vi "Image_processor.vi"(6 "DUT":u16, 9 "Ref Folder":path, 10 "DUT_Conf":string="RX-DUT", 11 "Image Path":path) -> (2 "Fail_Strings":string, 3 "PASS/FAIL":bool)   [LabVIEW 2024, in "Keyence_VS150.lvlib"]
uses:
  Keyence_VS150.lvlib
  Image_match_details.ctl
  <vilib>/Utility/file.llb/Read Delimited Spreadsheet (string).vi
  Launcher/Launcher_DTU.lvlib
panel:
  out "Array 3":T1[](array[typedef])
  out "Array 2":T1[](array[typedef])
  out "DUT":T2(plugin-control)
  out "Array":i32[](array[numeric])
  # "RY-DUT"
  # "RX-DUT"
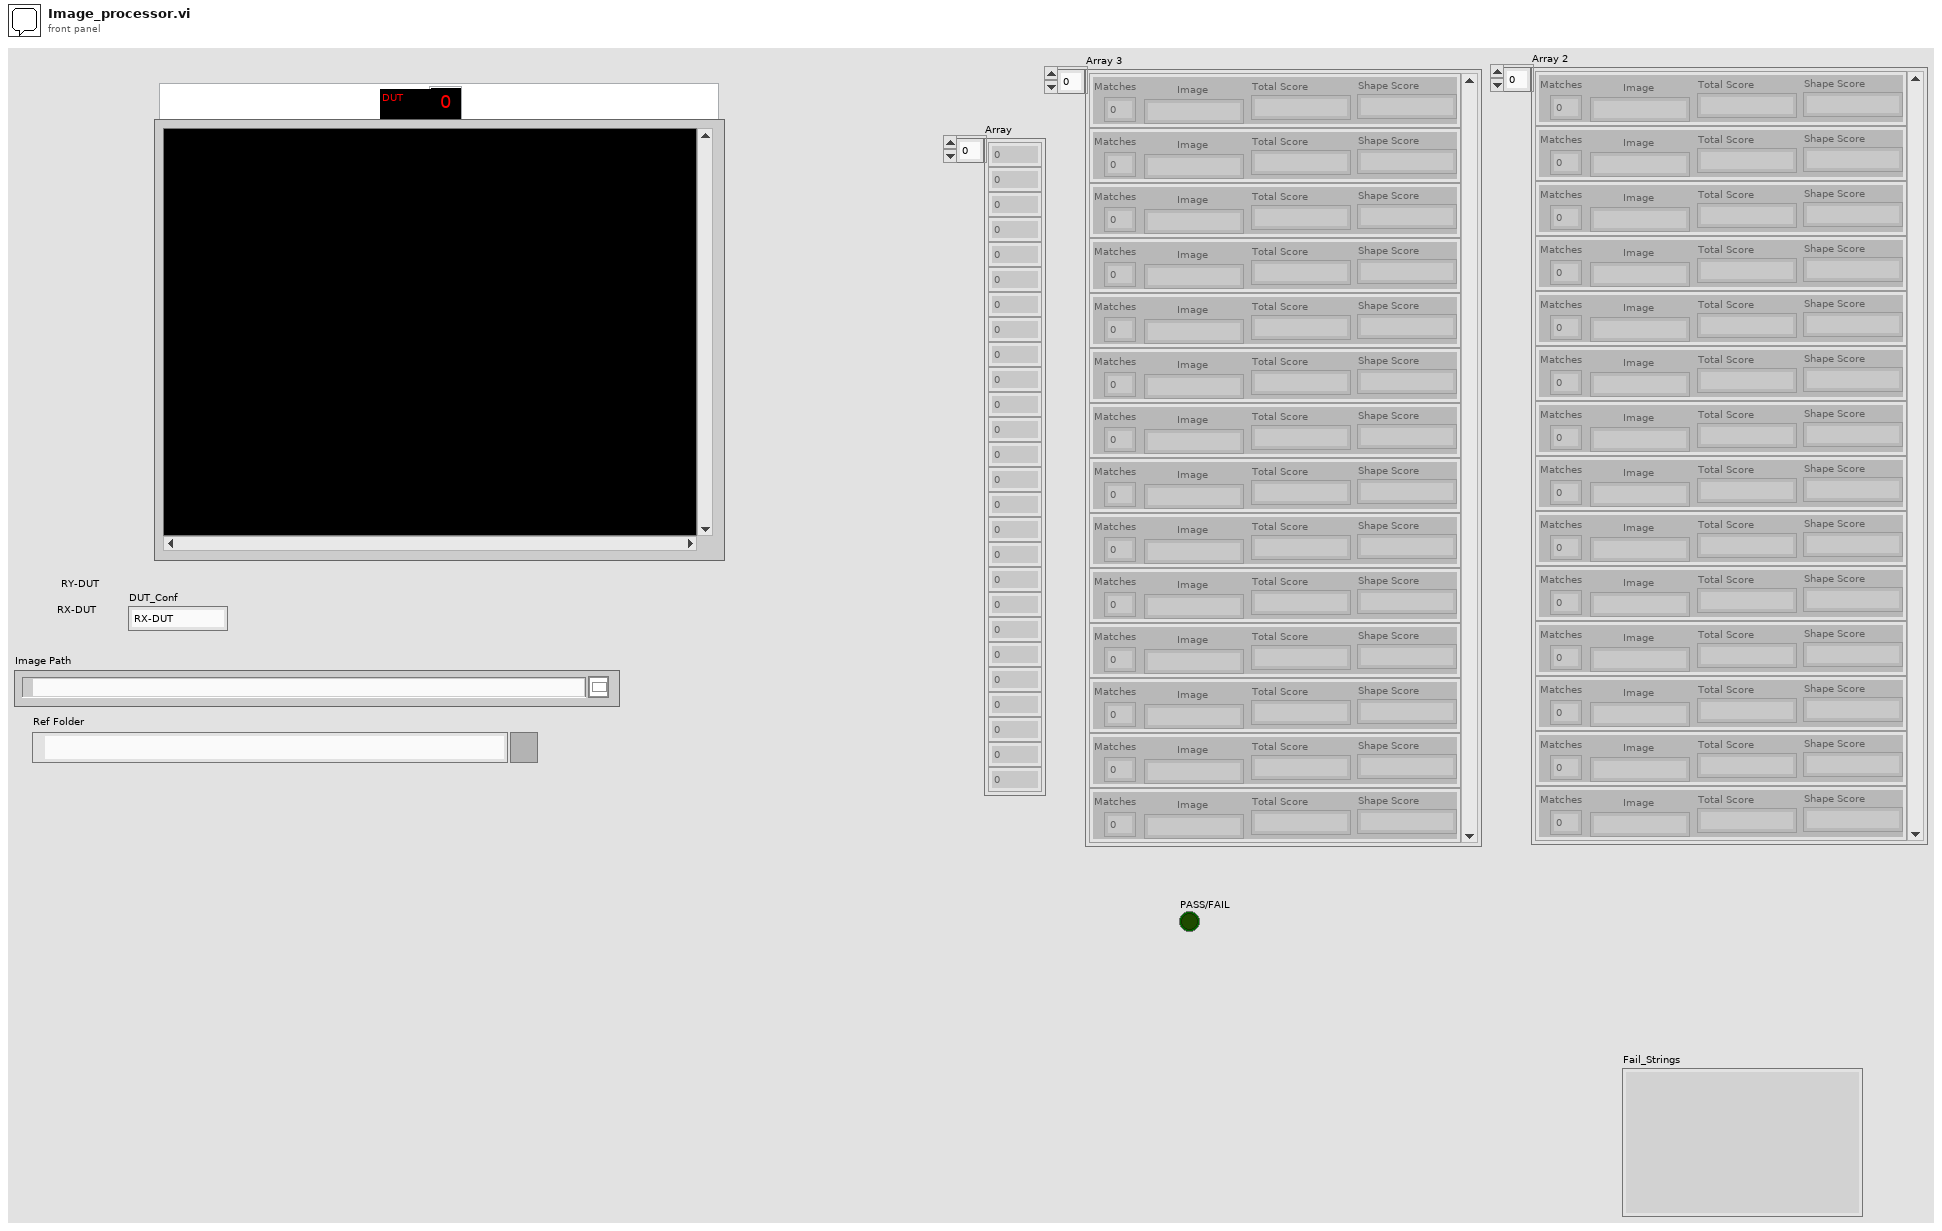
[diagram p1: front panel]
types:
  T1 = typedef "Image_match_details.ctl" = cluster{"Matches":i32, "Image":string, "Total Score":string, "Shape Score":string}
  T2 = typedef "IMAQ Image.ctl" = refnum<image>
  T3 = typedef "Image Type" = u32
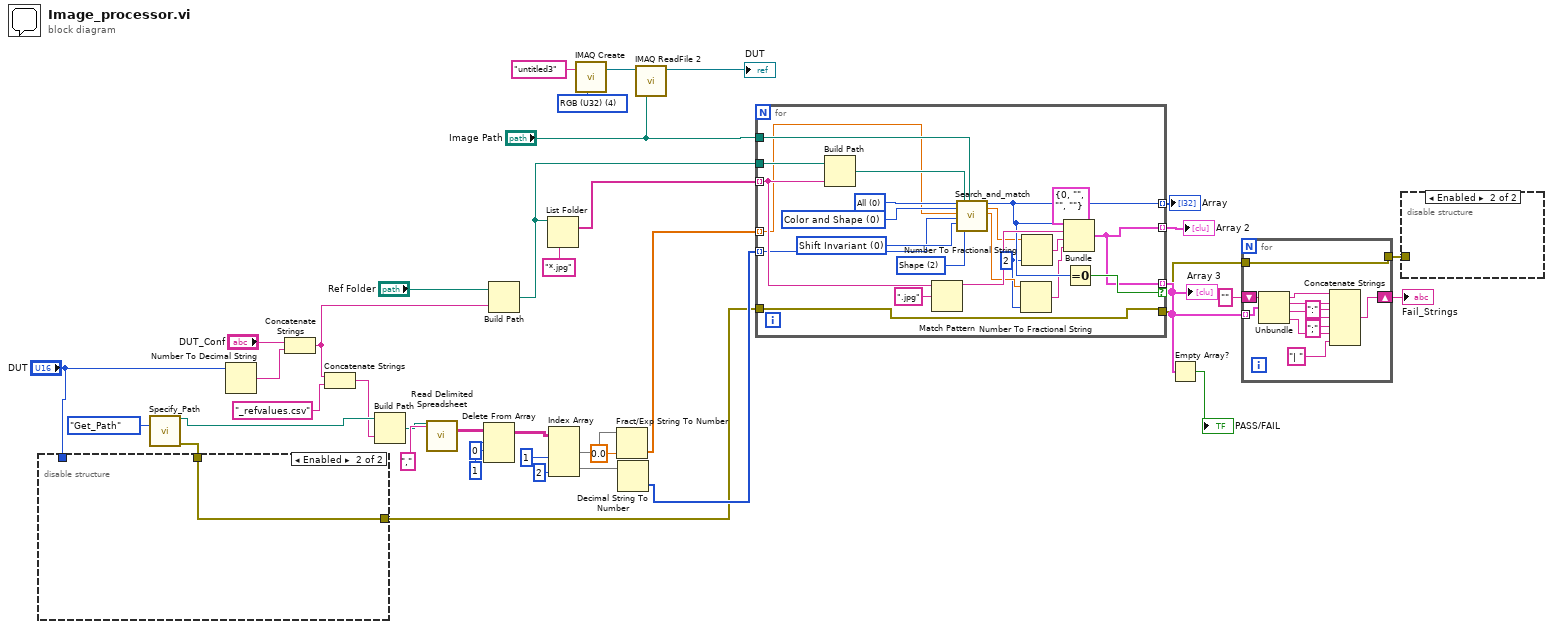
[diagram p0: block diagram]
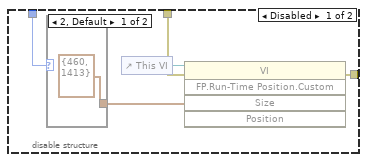
[diagram p2: hidden frame]
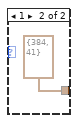
[diagram p3: hidden frame]
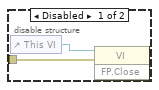
[diagram p4: hidden frame]
diagram:
  w11 = T3 4 items=["Grayscale (U8)", "Grayscale (I16)", "Grayscale (SGL)", "Complex (CSG)", "RGB (U32)", "HSL (U32)", "RGB (U64)", "Grayscale (U16)"] ("Image Type")
  n1 = call "Specify_Path.vi"("Path_Enum"=enum16{"Find_Path", "Get_Path"}."Get_Path") -> ("Configurations"=w21:path, "error out"=w6:errorcluster)  [unwired: 7 in, 6 out]
  n2 = disable-structure shown="Enabled" {
    disable-tunnel: w6 -> [w44 w48]
    disable-tunnel: "DUT" -> [w43 _]
    disable-tunnel: [w41 w48] -> w4
    frame Disabled {
      n3 = case shown="2, Default" w43 {
        tunnel: [cluster{"Top":i16, "Left":i16} {"Top"=460, "Left"=1413} ("Position") cluster{"Top":i16, "Left":i16} {"Top"=384, "Left"=41} ("Position")] -> w42
        frame 2, Default {
        }
        frame 1 {
        }
      }
      n4 = control-ref of="This VI"() -> (w45:refnum<vi>)
      n5 = invoke class="VI" method="FP.Run-Time Position.Custom"(reference=w45, error in=w44, "Size"=w42) -> (error out=w41:errorcluster)  [unwired: 2 in, 4 out]
    }
    frame Enabled {
    }
  }
  n6 = Number To Decimal String(number="DUT") -> (decimal integer string=w39:string)  [unwired: 1 in]
  n7 = Concatenate Strings("DUT_Conf", w39) -> (w23:string)
  n8 = Concatenate Strings(w23, "_refvalues.csv") -> (w20:string)
  n9 = Build Path(base path=w21, name or relative path=w20) -> (appended path=w19:path)
  n10 = call-poly <vilib>:"Read Delimited Spreadsheet.vi"("file path (dialog if empty)"=w19, "delimiter (\\t)"="," ("delimiter (\\t)")) -> ("all rows"=w32:string[][])  [unwired: 8 in, 5 out]
  n11 = Delete From Array(array=w32, length=1, index (row)=0) -> (array with subset deleted=w27:string[][])  [unwired: 1 in, 1 out]
  n12 = Build Path(base path="Ref Folder", name or relative path=w23) -> (appended path=w36:path)
  n13 = List Folder(path=w36, pattern="*.jpg") -> (filenames=w37:string[])  [unwired: 2 in, 3 out]
  n14 = Index Array(array=w27, index (col) #1=1 ("disabled index (col)"), index (col) #2=2 ("disabled index (col)")) -> (element #1=w29:string[], element #2=w28:string[])  [unwired: 2 in]
  n15 = call "IMAQ Create"("Image Name"="untitled3", "Image Type"=w11) -> ("New Image"=w9:T2)  [unwired: 3 in, 1 out]
  n16 = Fract/Exp String To Number(string=w29, default (0 dbl)=sgl 0.0 ("default (0 DBL)")) -> (number=w18:sgl[])  [unwired: 2 in, 1 out]
  n17 = Decimal String To Number(string=w28) -> (number=w17:i32[])  [unwired: 2 in, 1 out]
  n18 = call "IMAQ ReadFile 2"("File Path"="Image Path", "Image"=w9) -> ("Image Out"=→"DUT":T2)  [unwired: 5 in, 4 out]
  n19 = for {
    tunnel: w37 -> [w63] mode=indexing
    tunnel: w36 -> [w70]
    tunnel: "Image Path" -> [w68]
    tunnel: [w58] -> w35 mode=indexing
    tunnel: [w56] -> w1 mode=indexing
    tunnel: w18 -> [w60] mode=indexing
    tunnel: w17 -> [w59] mode=indexing
    tunnel: [w56] -> w13 mode=indexing if=w57
    tunnel: w4 -> [w53]
    tunnel: [w53] -> w3
    w51 = i16 2 ("precision (6)")
    w64 = u32 2 items=["Color and Shape", "Color", "Shape"] ("Match Feature Mode")
    w65 = u32 0 items=["Shift Invariant", "Rotation Invariant"] ("Match Mode")
    w66 = u32 0 items=["Color and Shape", "Color", "Shape "] ("Feature Mode")
    w67 = u32 0 items=["All", "Shift Information", "Rotation Information"] ("Learn Mode")
    n20 = Build Path(base path=w70, name or relative path=w63) -> (appended path=w69:path)
    n21 = Match Pattern(string=w63, regular expression=".jpg") -> (before substring=w61:string)  [unwired: 1 in, 3 out]
    n22 = call "Search_and_match.vi"("Learn Mode"=w67, "Feature Mode"=w66, "Minimum Match Score"=w60, "Number of Matches Requested"=w59, "Match Mode"=w65, "Ref path"=w69, "Match Feature Mode"=w64, "Main Path"=w68) -> ("Number of Matches"=w58:i32, "Total Score"=w55:sgl, "Shape Score"=w52:sgl)  [unwired: 9 in]
    n23 = Number To Fractional String(number=w52, precision (6)=w51) -> (F-format string=w50:string)  [unwired: 2 in]
    n24 = Number To Fractional String(number=w55, precision (6)=w51) -> (F-format string=w54:string)  [unwired: 2 in]
    n25 = Bundle(cluster=T1 {"Matches"=0, "Image"="", "Total Score"="", "Shape Score"=""} ("output cluster"), "Matches"=w58, "Image"=w61, "Total Score"=w54, "Shape Score"=w50) -> (w56:T1)
    n26 = Equal To 0?(x=w58) -> (x = 0?=w57:bool)
  }
  "Array" <- w35
  "Array 2" <- w1
  "Array 3" <- w13
  n27 = Empty Array?(array=w13) -> (empty?=→"PASS/FAIL":bool)
  n28 = for {
    tunnel: w13 -> [w80] mode=indexing
    shift-right: [w75] -> w14
    shift-left: "" -> [w74]
    tunnel: w3 -> [w73]
    tunnel: [w73] -> w2
    n29 = Unbundle(w80) -> ("Image"=w79:string, "Total Score"=w77:string, "Shape Score"=w71:string)  [unwired: 1 out]
    n30 = Concatenate Strings(w74, w79, ":" ("string"), w77, ";" ("string"), w71, "| " ("string")) -> (w75:string)
  }
  "Fail_Strings" <- w14
  n31 = disable-structure shown="Enabled" {
    disable-tunnel: w2 -> [w81 _]
    frame Disabled {
      n32 = control-ref of="This VI"() -> (w82:refnum<vi>)
      n33 = invoke class="VI" method="FP.Close"(reference=w82, error in=w81) -> ()  [unwired: 1 in, 3 out]
    }
    frame Enabled {
    }
  }
